vi "liszahárom.vi"() -> ()   [LabVIEW 2011]
panel:
  in  "stop":bool
  out "XY Graph":cluster{"Y":dbl[], "Y":dbl[]}[](graph)
  in  "fáziskülönbség":dbl
  in  "omegay":dbl
  in  "omega x":dbl
  in  "Ay":dbl
  in  "Ax":dbl
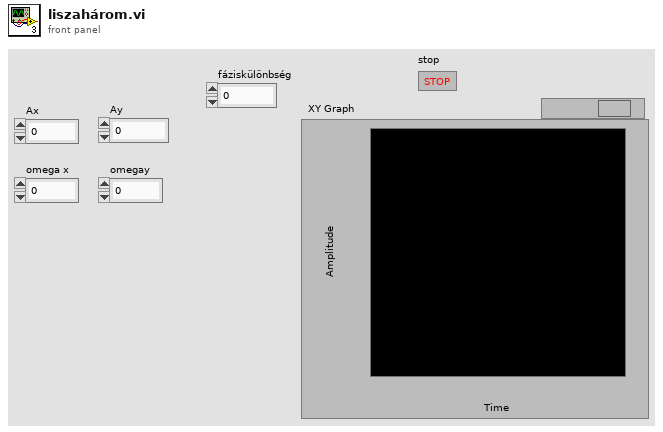
[diagram p1: front panel]
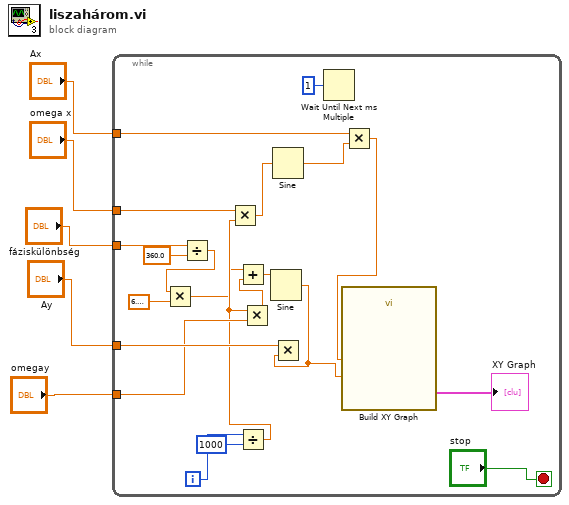
[diagram p0: block diagram]
diagram:
  n1 = while {
    tunnel: "Ax" -> [w24]
    tunnel: "omega x" -> [w20]
    tunnel: "Ay" -> [w17]
    tunnel: "omegay" -> [w15]
    tunnel: "fáziskülönbség" -> [w12]
    i -> [w22]
    stop <- "stop" stop-if-true
    n2 = Divide(x=w12, y=360.0) -> (x/y=w10:dbl)
    n3 = Multiply(x=w10, y=6.283185307179586) -> (x*y=w8:dbl)
    n4 = Divide(x=w22, y=1000) -> (x/y=w14:dbl)
    n5 = Multiply(x=w20, y=w14) -> (x*y=w19:dbl)
    n6 = Multiply(x=w14, y=w15) -> (x*y=w13:dbl)
    n7 = Add(x=w8, y=w13) -> (x+y=w7:dbl)
    n8 = Sine(x=w7) -> (sin(x)=w16:dbl)
    n9 = Sine(x=w19) -> (sin(x)=w23:dbl)
    n10 = Multiply(x=w17, y=w16) -> ()  [unwired: 1 out]
    n11 = Wait Until Next ms Multiple(millisecond multiple=u32 1) -> ()  [unwired: 1 out]
    n12 = Multiply(x=w24, y=w23) -> (x*y=w18:dbl)
    n13 = call "Build XY Graph"("Y Input"=w16, "X Input"=w18) -> ("XY Graph"=→"XY Graph":cluster{"Y":dbl[], "Y":dbl[]}[])  [unwired: 3 in, 6 out]
  }
